vi "rotationMatrix.vi"(3 "theta":dbl, 4 "Y":dbl[](array[numeric]), 5 "X":dbl[](array[numeric])) -> (0 "error":i32, 1 "Y Out":dbl[](array[numeric]), 2 "X Out":dbl[](array[numeric]))   [LabVIEW 2016]
uses:
  <vilib>/Analysis/coordinate.llb/2D Cartesian Coordinate Rotation (Array).vi
  <vilib>/Analysis/NI_AALPro.lvlib
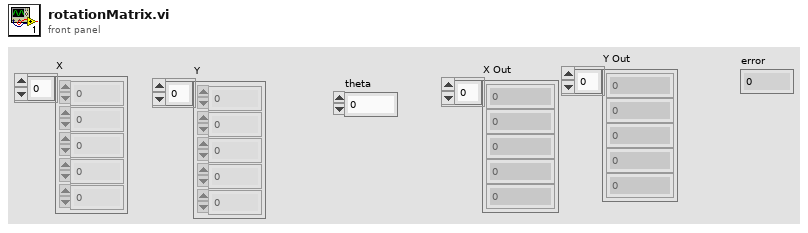
[diagram p1: front panel]
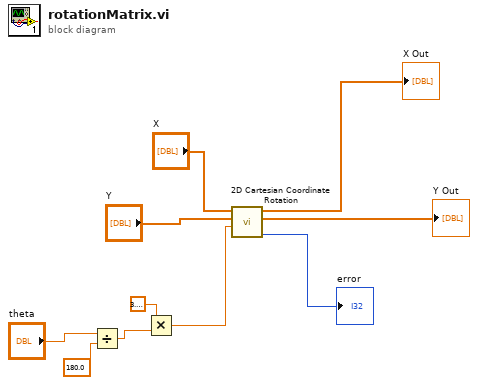
[diagram p0: block diagram]
diagram:
  n1 = Divide(x="theta", y=180.0) -> (x/y=w3:dbl)
  n2 = Multiply(x=3.141592653589793, y=w3) -> (x*y=w1:dbl)
  n3 = call-poly <vilib>:"2D Cartesian Coordinate Rotation.vi"("theta"=w1, "Y"="Y", "X"="X") -> ("error"=→"error":i32, "Y Out"=→"Y Out":dbl[], "X Out"=→"X Out":dbl[])  [unwired: 6 in]
